vi "Disconnect All Relays_v1.vi"(0 "TSM Context":T1, 11 "error in":errorcluster) -> (15 "error out":errorcluster)   [LabVIEW 2019]
uses:
  <vilib>/NI_TestStand_SemiconductorModule/NI_TestStand_Semiconductor_Module.lvlibp
  <vilib>/NI_TestStand_SemiconductorModule/NI_TestStand_Semiconductor_Module.lvlibp/PinMap/General/NIInstrumentTypeIDs.ctl
  <vilib>/NI_TestStand_SemiconductorModule/NI_TestStand_Semiconductor_Module.lvlibp/PinMap/Advanced/GetRelaysInRelayGroup.vi
  <vilib>/NI_TestStand_SemiconductorModule/NI_TestStand_Semiconductor_Module.lvlibp/1abvi3w/instr.lib/niSwitch/niswitch.llb/niSwitch Relay Action.ctl
  <vilib>/NI_TestStand_SemiconductorModule/NI_TestStand_Semiconductor_Module.lvlibp/PinMap/General/SemiconductorModuleContext.ctl
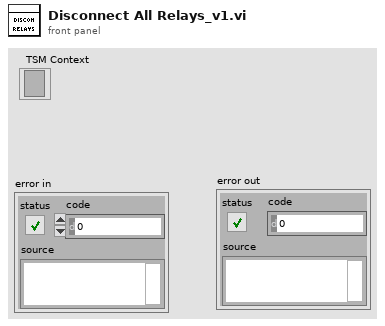
[diagram p1: front panel]
types:
  T1 = typedef "NI_TestStand_Semiconductor_Module.lvlibp/SemiconductorModuleContext.ctl" = refnum<k7>
  T2 = typedef "NI_TestStand_Semiconductor_Module.lvlibp/niSwitch Relay Action.ctl" = i32
  T3 = typedef "NI_TestStand_Semiconductor_Module.lvlibp/NIInstrumentTypeIDs.ctl" = string
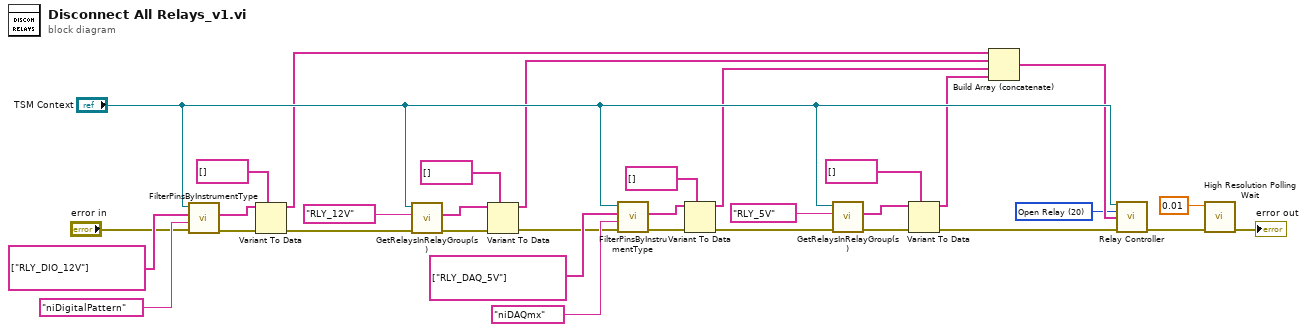
[diagram p0: block diagram]
diagram:
  w1 = T2 20 items=["Open Relay"=20, "Close Relay"=21] ("Relay Control")
  n1 = call <vilib>:"FilterPinsByInstrumentType.vi"("error in (no error)"="error in", "Instrument Type Id"=T3 "niDigitalPattern", "Pins"=tag[] ["RLY_DIO_12V"], "Semiconductor Module Context"="TSM Context") -> ("error out"=w29:errorcluster, "Filtered Pins"=w30:tag[])  [unwired: 5 in, 1 out]
  n2 = Variant To Data(error in=w29, type=string[] [] ("Relay Resource Names"), Variant=w30) -> (data=w9:string[], error out=w26:errorcluster)
  n3 = call-poly <vilib>:"GetRelaysInRelayGroup(s).vi"("error in (no error)"=w26, "Relay Group"=tag "RLY_12V", "Semiconductor Module Context"="TSM Context") -> ("error out"=w24:errorcluster, "Relays"=w25:tag[])  [unwired: 6 in, 1 out]
  n4 = Variant To Data(error in=w24, type=string[] [] ("Relay Resource Names"), Variant=w25) -> (data=w8:string[], error out=w12:errorcluster)
  n5 = call <vilib>:"FilterPinsByInstrumentType.vi"("error in (no error)"=w12, "Instrument Type Id"=T3 "niDAQmx", "Pins"=tag[] ["RLY_DAQ_5V"], "Semiconductor Module Context"="TSM Context") -> ("error out"=w18:errorcluster, "Filtered Pins"=w19:tag[])  [unwired: 5 in, 1 out]
  n6 = Variant To Data(error in=w18, type=string[] [] ("Relay Resource Names"), Variant=w19) -> (data=w7:string[], error out=w13:errorcluster)
  n7 = call-poly <vilib>:"GetRelaysInRelayGroup(s).vi"("error in (no error)"=w13, "Relay Group"=tag "RLY_5V", "Semiconductor Module Context"="TSM Context") -> ("error out"=w14:errorcluster, "Relays"=w15:tag[])  [unwired: 6 in, 1 out]
  n8 = Variant To Data(error in=w14, type=string[] [] ("Relay Resource Names"), Variant=w15) -> (data=w6:string[], error out=w11:errorcluster)
  n9 = Build Array (concatenate)(w9, w8, w7, w6) -> (w5:string[])
  n10 = call "Relay Controller.vi"("TSM Context"="TSM Context", 5:w1, "Relays"=w5, "error in"=w11) -> ("error out"=w3:errorcluster)  [unwired: 11 in]
  n11 = call <vilib>:"High Resolution Polling Wait.vi"("error in (no error)"=w3, "seconds to wait"=0.01) -> ("error out"=→"error out":errorcluster)  [unwired: 9 in]
